vi "Run Test.vi"(8 "error in (no error)":errorcluster, 11 "Test Template in":refnum<class "LCM Single-Up Post-Flash Test.lvclass">) -> (0 "error out":errorcluster, 1 "Fail Codes":string[](array[string]), 2 "Tests Passed":bool[](array[boolean]), 3 "Test Template out":refnum<class "LCM Single-Up Post-Flash Test.lvclass">)   [LabVIEW 2015, in "LCM Single-Up Post-Flash Test.lvclass"]
uses:
  LCM Single-Up Post-Flash Test.lvclass
  LCM Single-Up Power Up/LCM Single-Up Power Up.lvclass
  Test Class/Test Class.lvclass
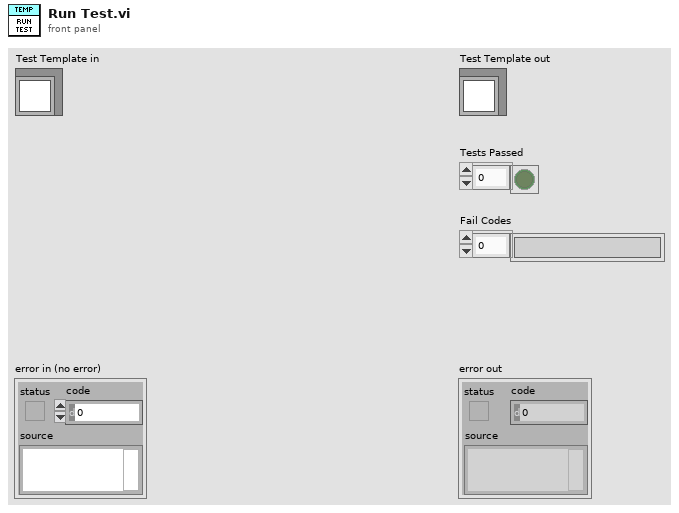
[diagram p1: front panel]
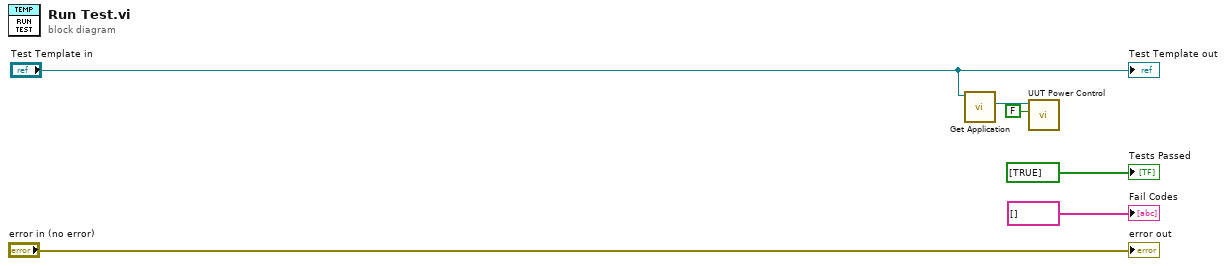
[diagram p0: block diagram]
diagram:
  n1 = call "Get Application.vi"("Test Class in"="Test Template in") -> ("Application.lvlib:Application.lvclass"=w2:refnum<class "Application.lvclass">)  [unwired: 9 in, 1 out]
  n2 = call "UUT Power Control.vi"("Connect (False)"=FALSE, "Application in"=w2) -> ()  [unwired: 9 in, 1 out]
  "error out" <- "error in (no error)"
  "Test Template out" <- "Test Template in"
  "Tests Passed" <- bool[] [TRUE] ("Tests Passed")
  "Fail Codes" <- string[] [] ("Fail Codes")
